vi "Read circulationVelocity.vi"(8 "error in (no error)":errorcluster, 11 "CirculateSkill in":refnum<class "CirculateSkill.lvclass">) -> (0 "error out":errorcluster, 2 "circulationVelocity":dbl, 3 "CirculateSkill out":refnum<class "CirculateSkill.lvclass">)   [LabVIEW 2022 SP3, in "CirculateSkill.lvclass"]
uses:
  CirculateSkill.lvclass
  CirculateSkill.lvclass/CirculateSkill.ctl
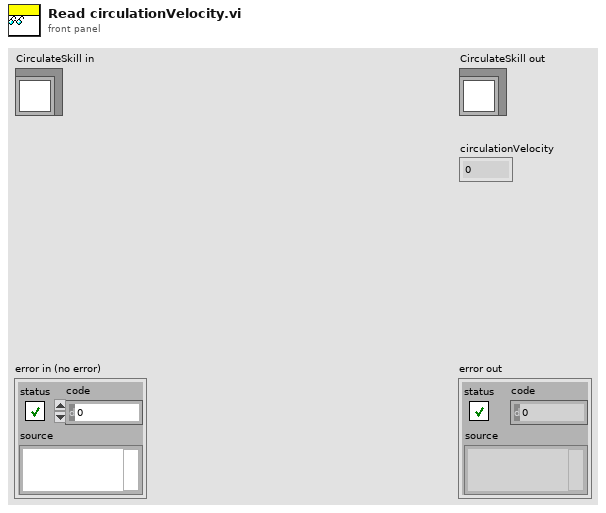
[diagram p1: front panel]
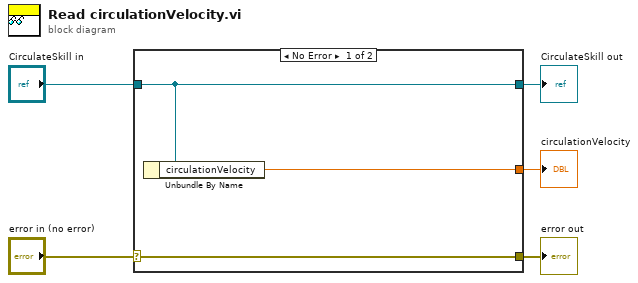
[diagram p0: block diagram]
diagram:
  n1 = case shown="No Error" "error in (no error)" {
    selector: "error in (no error)" -> [w8 w9]
    tunnel: [w8 w9] -> w4
    tunnel: [w7 w10] -> w2
    tunnel: "CirculateSkill in" -> [w7 w10]
    tunnel: [w6 _] -> w1
    frame No Error {
      n2 = Unbundle By Name(w7) -> ("circulationVelocity"=w6:dbl)
    }
    frame Error {
    }
  }
  "error out" <- w4
  "CirculateSkill out" <- w2
  "circulationVelocity" <- w1
